vi "Com_SECS Equipment _Data Message_Character.vi"(7 "Parent Index":i32=-1, 8 "error in":errorcluster, 10 "Data":string, 11 "Message Data In":T1[](array[typedef])) -> (0 "error out":errorcluster, 3 "Message Data Out":T1[](array[typedef]))   [LabVIEW 2016]
uses:
  Data Def/Com_SECS Equipment _Message Data.ctl
  Data Def/Com_SECS Equipment _Data Item Format.ctl
  Data Def/Com_SECS Equipment _Format Code.ctl
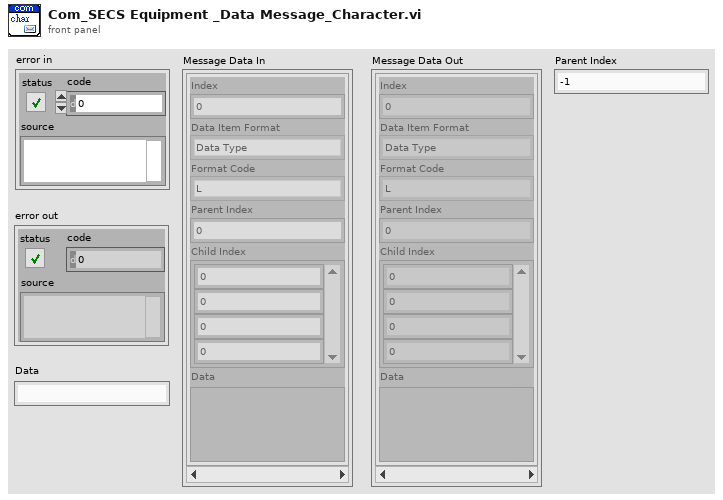
[diagram p1: front panel]
types:
  T1 = typedef "Com_SECS Equipment _Message Data.ctl" = cluster{"Index":i32, "Data Item Format":T2, "Format Code":T3, "Parent Index":i32, "Child Index":i32[], "Data":variant}
  T2 = typedef "Com_SECS Equipment _Data Item Format.ctl" = enum16{"Data Type", "Value"}
  T3 = typedef "Com_SECS Equipment _Format Code.ctl" = enum16{"L", "A", "B", "Boolean", "J", "I1", "I2", "I4", "I8", "U1", "U2", "U4", "U8", "F4", "F8", "Char"}
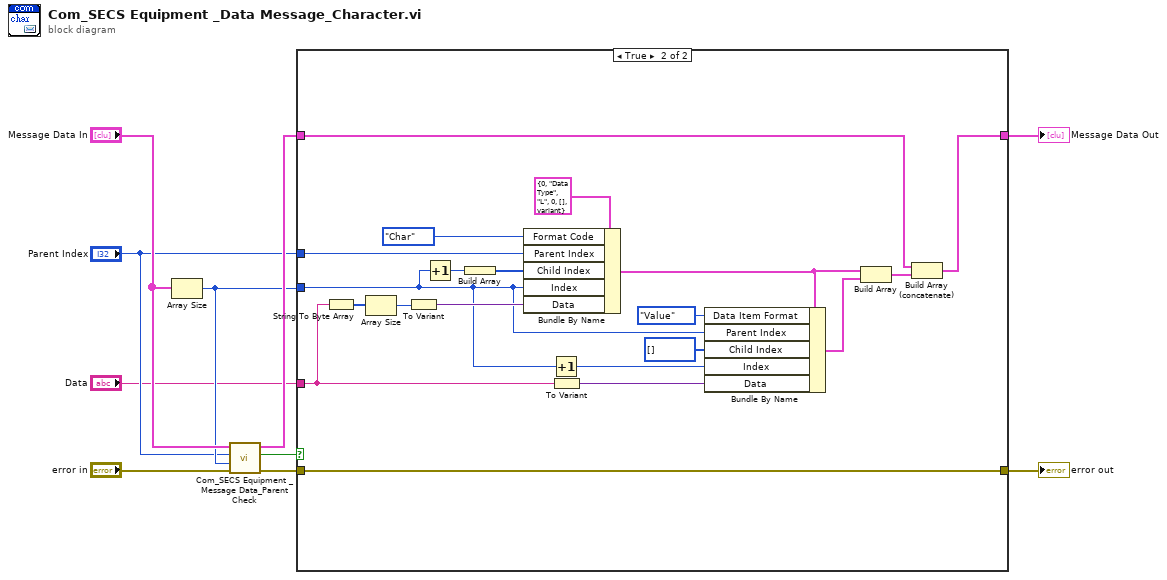
[diagram p0: block diagram]
diagram:
  n1 = Array Size(array="Message Data In") -> (size(s)=w5:i32)
  n2 = call "Com_SECS Equipment _Message Data_Parent Check.vi"("error in"="error in", "Message Index"=w5, "Parent Index"="Parent Index", "Message Data In"="Message Data In") -> ("error out"=w8:errorcluster, "OK?"=w9:bool, "Message Data Out"=w6:T1[])  [unwired: 5 in]
  n3 = case shown="True" w9 {
    tunnel: w8 -> [w11 w16]
    tunnel: w6 -> [w12 w18]
    tunnel: [w12 w17] -> w4
    tunnel: "Parent Index" -> [_ w25]
    tunnel: w5 -> [_ w15]
    tunnel: "Data" -> [_ w14]
    tunnel: [w11 w16] -> w3
    frame False {
    }
    frame True {
      n4 = String To Byte Array(string=w14) -> (unsigned byte array=w13:u8[])
      n5 = Array Size(array=w13) -> (size(s)=w28:i32)
      n6 = To Variant(anything=w28) -> (Variant=w27:variant)
      n7 = Increment(x=w15) -> (x+1=w30:i32)
      n8 = Build Array(w30) -> (w29:i32[])
      n9 = Bundle By Name(cluster=T1 {"Index"=0, "Data Item Format"=enum."Data Type", "Format Code"=enum."L", "Parent Index"=0, "Child Index"=[], "Data"=variant} ("Message Data"), "Format Code"=Com_SECS_Equipment__Format_Code."Char", "Parent Index"=w25, "Child Index"=w29, "Index"=w15, "Data"=w27) -> (w21:T1)
      n10 = Increment(x=w15) -> (x+1=w23:i32)
      n11 = To Variant(anything=w14) -> (Variant=w22:variant)
      n12 = Bundle By Name(cluster=w21, "Data Item Format"=Com_SECS_Equipment__Data_Item_Format."Value", "Parent Index"=w15, "Child Index"=i32[] [], "Index"=w23, "Data"=w22) -> (w20:T1)
      n13 = Build Array(w21, w20) -> (w19:T1[])
      n14 = Build Array (concatenate)(w18, w19) -> (w17:T1[])
    }
  }
  "error out" <- w3
  "Message Data Out" <- w4
